vi "isConnected.vi"(8 "error in (no error)":errorcluster, 11 "Client in":refnum<class "Client.lvclass">) -> (0 "error out":errorcluster, 2 "connected":bool, 3 "Client out":refnum<class "Client.lvclass">)   [LabVIEW 2013, in "MQTT Client.lvlib" / "Client.lvclass"]
uses:
  Client.lvclass
  Client.lvclass/Client.ctl
  <vilib>/LabVIEW Open Source Project/MQTT Connection/MQTT_Base/Session/Session.lvclass
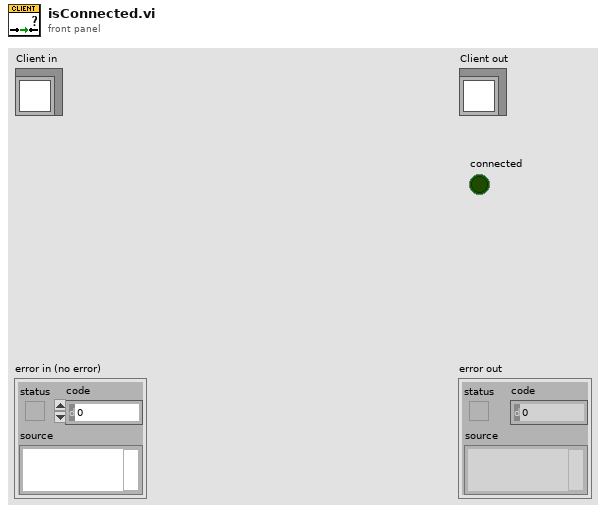
[diagram p1: front panel]
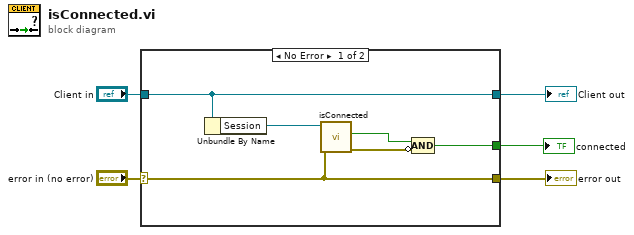
[diagram p0: block diagram]
diagram:
  n1 = case shown="No Error" "error in (no error)" {
    selector: "error in (no error)" -> [w9 w13]
    tunnel: [w9 w13] -> w4
    tunnel: [w11 w12] -> w2
    tunnel: "Client in" -> [w11 w12]
    tunnel: [w6 _] -> w1
    frame No Error {
      n2 = Unbundle By Name(w11) -> ("Session"=w10:refnum<class "Session.Client.lvclass">)
      n3 = call <vilib>:"isConnected.vi"("error in (no error)"=w9, "Session in"=w10) -> ("error out"=w8:errorcluster, "connected"=w7:bool)  [unwired: 7 in, 1 out]
      n4 = Compound Arithmetic op=AND(w7, invert w8) -> (w6:bool)
    }
    frame Error {
    }
  }
  "error out" <- w4
  "Client out" <- w2
  "connected" <- w1
